vi "SPAM-ExtCmd.vi"() -> ()   [LabVIEW 2010]
panel:
  out "CID":refnum<k5>
  in  "Mode":u16(ring) items=["telinfo", "teloffset aléatoire"]
  in  "Composite ?":bool
  out "error out":errorcluster
  in  "quit":bool
  in  "connect":bool
  out "Cx":bool
  in  "Port":u16=8181
  in  "address":string="132.204.61.34" caption="Adresse de BonOMM"
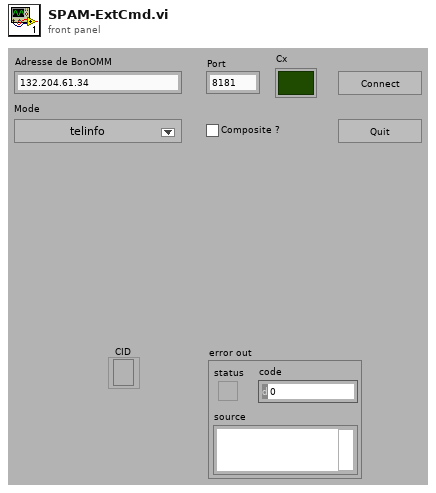
[diagram p1: front panel]
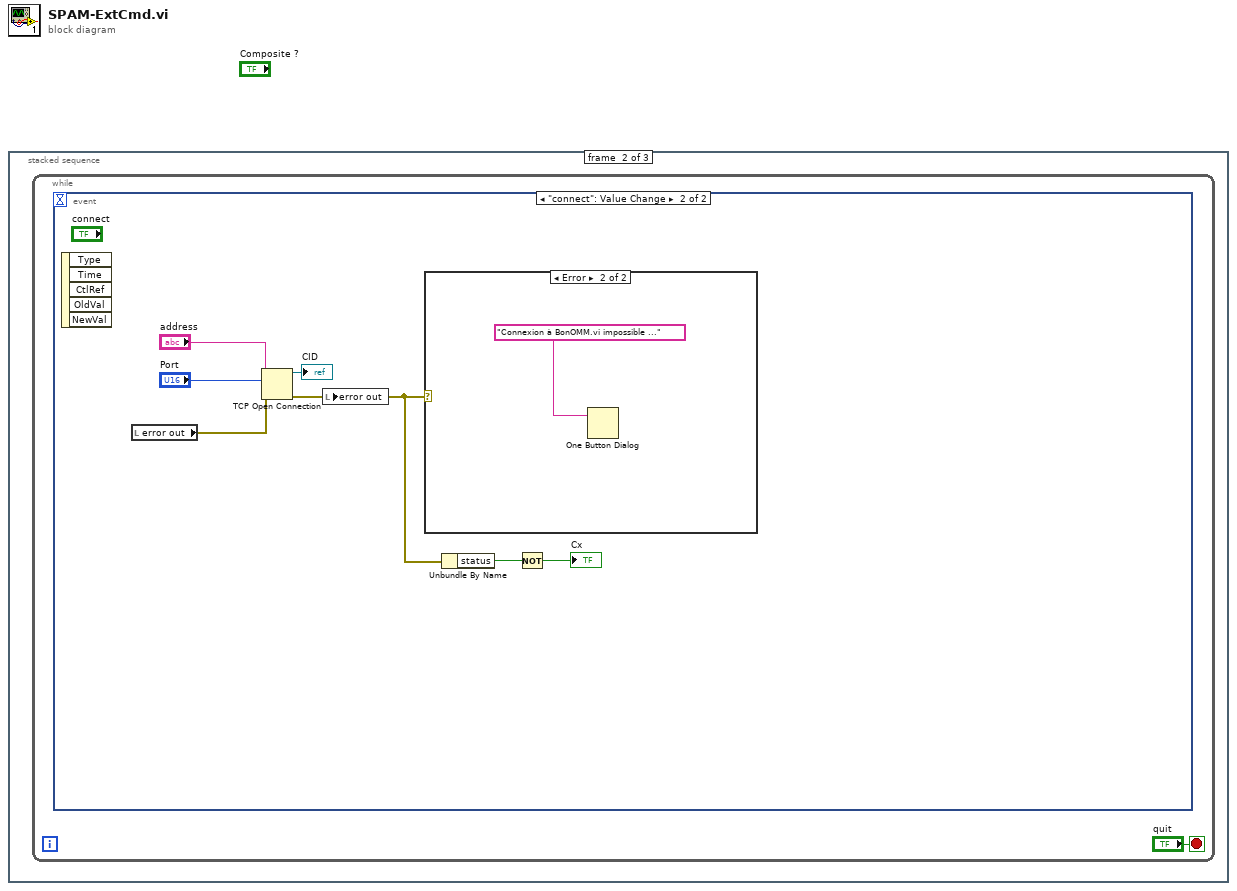
[diagram p0: block diagram]
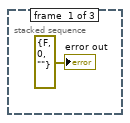
[diagram p2: hidden frame]
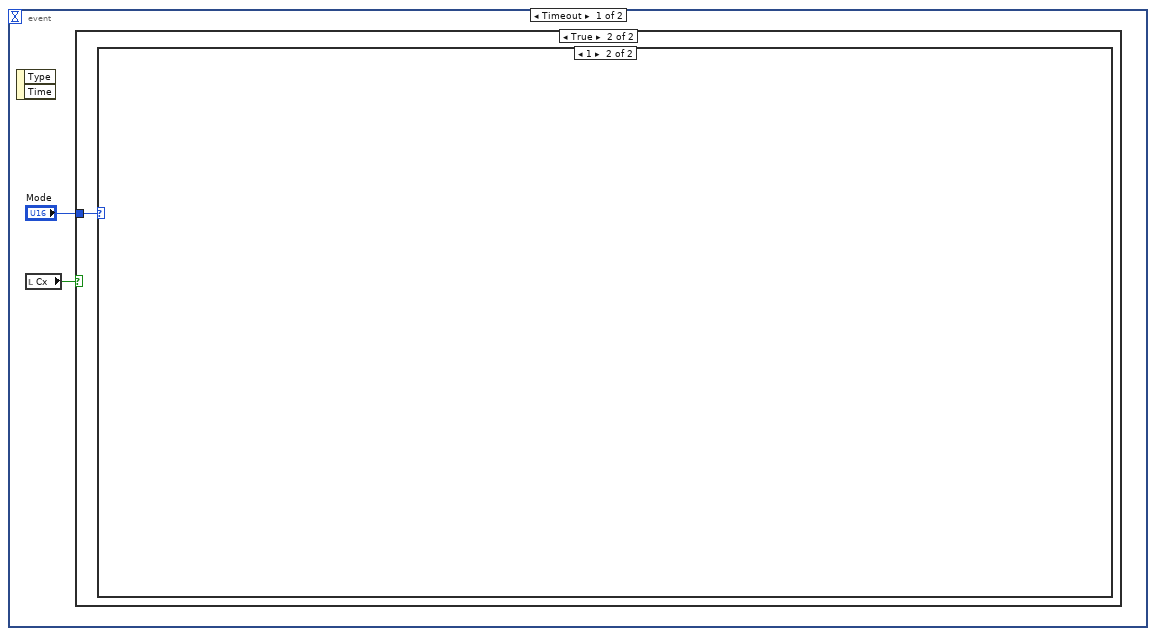
[diagram p3: hidden frame]
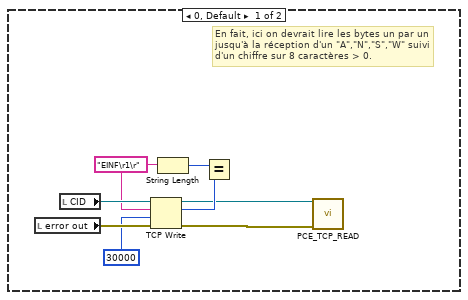
[diagram p5: hidden frame]
diagram:
  n1 = stacked-sequence {
    frame #0 {
      "error out" <- errorcluster {"status"=FALSE, "code"=0, "source"=""} ("error out")
    }
    frame #1 {
      n2 = while {
        stop <- "quit" stop-if-true
        n3 = event shown="[1] \"connect\": Value Change" {
          selector: _ -> [_ _]
          dyn-events: _ -> [_ _]
          timeout: _ -> [_ _]
          event Timeout {
            n4 = event-data() -> ()  [unwired: 1 in, 2 out]
            n5 = local read "Cx"() -> (w4:bool)
            n6 = case shown="True" w4 {
              tunnel: "Mode" -> [_ w5]
              frame False {
              }
              frame True {
                n7 = case shown="1" w5 {
                  frame 0, Default {
                    w9 = "EINF\r1\r" ("data in")
                    # "En fait, ici on devrait lire les bytes un par un\njusqu'à la réception d'un \"A\",\"N\",\"S\",\"W\" suivi\nd'un chiffre sur 8 caractères > 0."
                    n8 = local read "error out"() -> (w12:errorcluster)
                    n9 = local read "CID"() -> (w13:refnum<k5>)
                    n10 = TCP Write(connection ID=w13, data in=w9, error in (no error)=w12, 9:30000 ("timeout ms (25000)")) -> (connection ID out=w7:refnum<k5>, bytes written=w10:i32, error out=w6:errorcluster)
                    n11 = String Length(string=w9) -> (length=w8:i32)
                    n12 = Equal?(x=w8, y=w10) -> ()  [unwired: 1 out]
                    n13 = call "PCE_TCP_READ.vi"("ConnID IN"=w7, "Error IN"=w6) -> ()  [unwired: 11 in, 3 out]
                  }
                  frame 1 {
                  }
                }
              }
            }
          }
          event "connect": Value Change {
            n14 = event-data() -> ()  [unwired: 1 in, 5 out]
            n15 = local read "error out"() -> (w18:errorcluster)
            n16 = TCP Open Connection(address="address", remote port or service name="Port", error in (no error)=w18) -> (connection ID=→"CID":refnum<k5>, error out=w17:errorcluster)  [unwired: 2 in]
            n17 = local write "error out"(w17) -> ()
            n18 = case shown="Error" w17 {
              frame No Error {
              }
              frame Error {
                n19 = One Button Dialog(message="Connexion à BonOMM.vi impossible ...") -> ()  [unwired: 1 in, 1 out]
              }
            }
            n20 = Unbundle By Name(w17) -> ("status"=w16:bool)
            n21 = Not(x=w16) -> (.not. x?=→"Cx":bool)
          }
        }
      }
    }
    frame #2 {
    }
  }
